vi "Ion Gauge Monitor.vi"() -> ()   [LabVIEW 2014]
uses:
  <vilib>/Instr/_visa.llb/VISA Configure Serial Port (Instr).vi
panel:
  out "SAES IP Pressure":string
  out "Current Pressure":dbl
  in  "stop":bool
  out "Pressure of Ion Gauge":waveform(dbl)(graph)
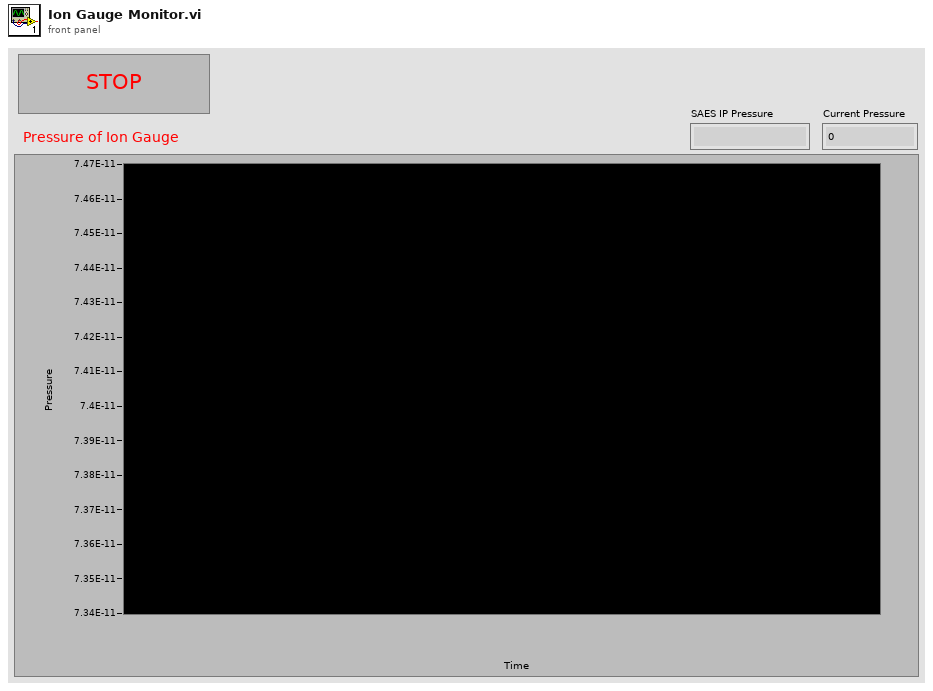
[diagram p1: front panel]
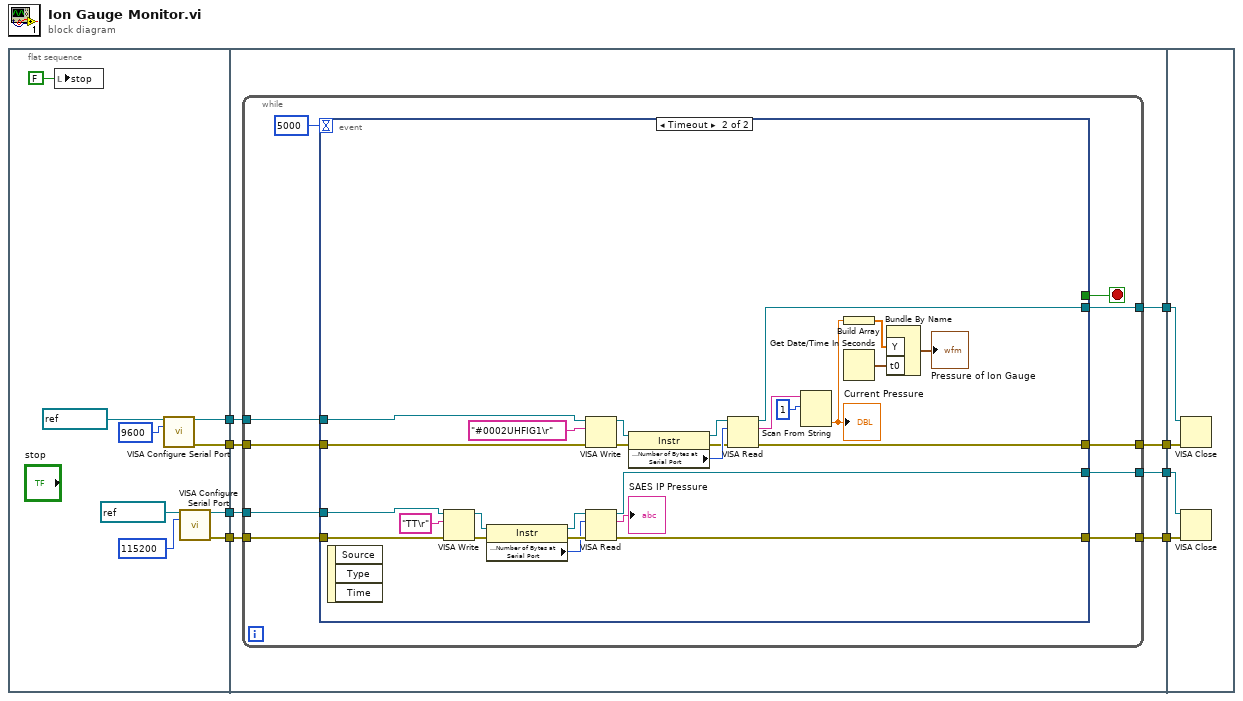
[diagram p0: block diagram]
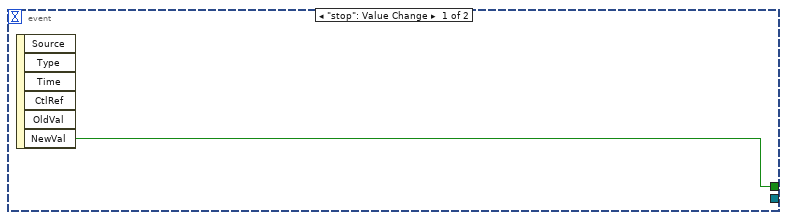
[diagram p2: hidden frame]
diagram:
  n1 = flat-sequence {
    tunnel: [w14] -> w4
    tunnel: [w13] -> w3
    tunnel: [w11] -> w2
    tunnel: [w10] -> w1
    tunnel: [w25] -> w8
    tunnel: [w24] -> w7
    tunnel: [w23] -> w6
    tunnel: [w22] -> w5
    tunnel: w4 -> [w21]
    tunnel: w3 -> [w20]
    tunnel: w2 -> [w19]
    tunnel: w1 -> [w18]
    tunnel: w8 -> [w67]
    tunnel: w7 -> [w66]
    tunnel: w6 -> [w65]
    tunnel: w5 -> [w64]
    frame #0 {
      n2 = local write "stop"(FALSE ("stop")) -> ()
      n3 = call-poly "VISA Configure Serial Port"("VISA resource name"=refnum<visa-resource-name> "COM4", "baud rate (9600)"=u32 9600) -> ("VISA resource name out"=w11:refnum<visa-resource-name>, "error out"=w10:errorcluster)  [unwired: 12 in]
      n4 = call-poly "VISA Configure Serial Port"("VISA resource name"=refnum<visa-resource-name> "COM9", "baud rate (9600)"=u32 115200) -> ("VISA resource name out"=w13:refnum<visa-resource-name>, "error out"=w14:errorcluster)  [unwired: 12 in]
    }
    frame #1 {
      n5 = while {
        tunnel: [w29] -> w25
        tunnel: [w30] -> w24
        tunnel: w20 -> [w32]
        tunnel: w21 -> [w31]
        tunnel: [w27] -> w22
        tunnel: [w28] -> w23
        tunnel: w19 -> [w34]
        tunnel: w18 -> [w33]
        stop <- w35 stop-if-true
        n6 = event shown="[1] Timeout" {
          selector: _ -> [_ _]
          dyn-events: _ -> [_ _]
          timeout: 5000 -> [_ _]
          tunnel: [w36 _] -> w35
          tunnel: w34 -> [_ w44]
          tunnel: w33 -> [_ w43]
          tunnel: w32 -> [_ w42]
          tunnel: w31 -> [_ w41]
          tunnel: [_ w40] -> w30
          tunnel: [_ w39] -> w29
          tunnel: [_ w38] -> w28
          tunnel: [_ w37] -> w27
          event "stop": Value Change {
            n7 = event-data() -> ("NewVal"=w36:bool)  [unwired: 1 in, 5 out]
          }
          event Timeout {
            n8 = event-data() -> ()  [unwired: 1 in, 3 out]
            n9 = VISA Write(VISA resource name=w42, write buffer="TT\r", error in (no error)=w41) -> (VISA resource name out=w48:refnum<visa-resource-name>, error out=w50:errorcluster)  [unwired: 1 out]
            n10 = property class="Instr"(reference=w48, error in=w50) -> (reference out=w49:refnum<visa-resource-name>, error out=w58:errorcluster, "Serial Settings:Number of Bytes at Serial Port"=w51:u32)
            n11 = VISA Write(VISA resource name=w44, write buffer="#0002UHFIG1\r", error in (no error)=w43) -> (VISA resource name out=w61:refnum<visa-resource-name>, error out=w59:errorcluster)  [unwired: 1 out]
            n12 = VISA Read(VISA resource name=w49, byte count=w51, error in (no error)=w58) -> (VISA resource name out=w38:refnum<visa-resource-name>, read buffer=→"SAES IP Pressure":string, error out=w37:errorcluster)  [unwired: 1 out]
            n13 = property class="Instr"(reference=w61, error in=w59) -> (reference out=w62:refnum<visa-resource-name>, error out=w60:errorcluster, "Serial Settings:Number of Bytes at Serial Port"=w63:u32)
            n14 = VISA Read(VISA resource name=w62, byte count=w63, error in (no error)=w60) -> (VISA resource name out=w39:refnum<visa-resource-name>, read buffer=w46:string, error out=w40:errorcluster)  [unwired: 1 out]
            n15 = Scan From String(input string=w46, initial scan location=u32 1) -> (output 1=w57:dbl)  [unwired: 3 in, 3 out]
            "Current Pressure" <- w57
            n16 = Build Array(w57) -> (w56:dbl[])
            n17 = Get Date/Time In Seconds() -> (seconds since 1Jan1904=w54:timestamp)
            n18 = Bundle By Name("Y"=w56, "t0"=w54) -> (→"Pressure of Ion Gauge":waveform(dbl))  [unwired: 1 in]
          }
        }
      }
    }
    frame #2 {
      n19 = VISA Close(VISA resource name=w67, error in (no error)=w66) -> ()  [unwired: 1 out]
      n20 = VISA Close(VISA resource name=w65, error in (no error)=w64) -> ()  [unwired: 1 out]
    }
  }
